vi "Periodic Sinc Pattern.vi"(7 "delay (s)":dbl, 8 "delta t (s)":dbl=0.1, 9 "order":i32=9, 10 "amplitude":dbl=1.0, 11 "samples":i32=128) -> (0 "error":i32, 3 "Periodic Sinc Pattern":dbl[](array[numeric]))   [LabVIEW 2024, in "NI_AALBase.lvlib"]
doc: "<p>Generates an array containing a periodic sinc pattern.</p>"
uses:
  NI_AALBase.lvlib
panel:
  # "Periodic Sinc Pattern"
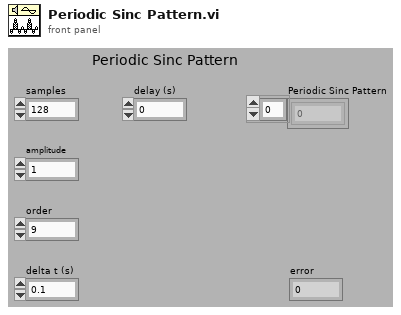
[diagram p1: front panel]
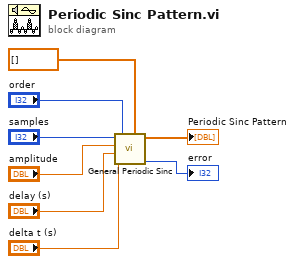
[diagram p0: block diagram]
diagram:
  n1 = call "General Periodic Sinc.vi"("X"=dbl[] [], "n"="order", "delta t"="delta t (s)", "delay"="delay (s)", "amplitude"="amplitude", "samples"="samples") -> ("error"=→"error":i32, "Periodic Sinc Pattern"=→"Periodic Sinc Pattern":dbl[])  [unwired: 4 in]
